vi "Write Result.vi"(0 "Charact Result Accessor in":refnum<class "Charact Result Accessor.lvclass">, 5 "Charact Result":variant, 11 "error in":errorcluster) -> (4 "Charact Result Accessor out":refnum<class "Charact Result Accessor.lvclass">, 15 "error out":errorcluster)   [LabVIEW 2023, in "RFFixtureCharact.RFPM.lvlib" / "Charact Result Accessor.lvclass"]
uses:
  Charact Result Accessor.lvclass
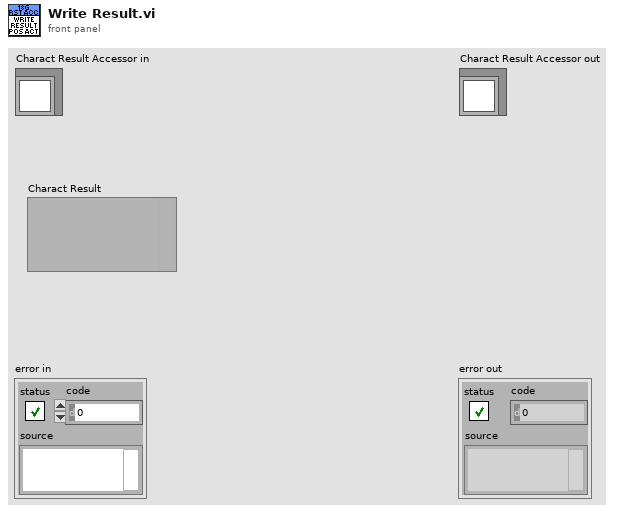
[diagram p1: front panel]
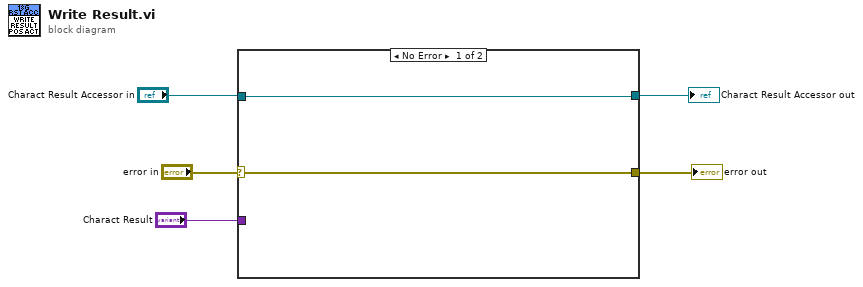
[diagram p0: block diagram]
diagram:
  n1 = case shown="No Error" "error in" {
    selector: "error in" -> [w7 w9]
    tunnel: [w7 w9] -> w4
    tunnel: "Charact Result Accessor in" -> [w6 w8]
    tunnel: [w6 w8] -> w2
    tunnel: "Charact Result" -> [_ _]
    frame No Error {
    }
    frame Error {
    }
  }
  "error out" <- w4
  "Charact Result Accessor out" <- w2
